vi "AR Example.vi"() -> ()   [LabVIEW 2020]
uses:
  UI_Actor/UI_Actor/ctl_AR_Parameters.ctl
  UI_Actor/UI_Actor/ctl_AR_Mode.ctl
  UIA_ChildTest/UIA_ChildTest/UIA_ChildTest.lvclass
  D:/Projets/STEP AT/UI Actor/UI_Actor/UI_Actor/UI_Actor.lvclass
  UI_Actor/UI_Actor Messages/UI_ShowIn_FreeWindow Msg/UI_ShowIn_FreeWindow Msg.lvclass/UI_ShowIn_FreeWindow Msg.ctl
  UI_Actor/UI_Actor Messages/UI_AutoRefresh Msg/UI_AutoRefresh Msg.lvclass/UI_AutoRefresh Msg.ctl
  support/Actor Framework.lvlibp/Message Enqueuer/Enqueue.vi
  UI_Actor/UI_Actor Messages/UI_ShowIn_FreeWindow Msg/UI_ShowIn_FreeWindow Msg.lvclass
  UI_Actor/UI_Actor Messages/UI_AutoRefresh Msg/UI_AutoRefresh Msg.lvclass
  UI_Actor/UI_Actor/UI_Actor.lvclass
  support/Actor Framework.lvlibp/Stop Msg/Stop Msg.lvclass
  support/Databox.lvlibp
panel:
  in  "Data":dbl[](array[numeric])=[2.0, 2.0, 5.0, 0.0, 0.0, 0.0, 0.0, 3.0, 0.0]
  in  "Parameters":T1={"Write TipStrips with details (T)"=TRUE, "Write Captions with UserLabels (T)"=TRUE, "Mode (ind only)"=enum."Indicators only", "Enable nested stream (T)"=TRUE}
  in  "Units":string[](array[string])=["%", "km", "°C", "-", "", "", " ", "kV", "A"]
  in  "UserLab":string[](array[string])=["coucou 1", "coucou 2", "temp", "c chaud", "", "", " ", "yes!", "Clust num"]
  in  "SysLab":string[](array[string])=["Ctl1", "Ctl2", "indic1", "indic2", "ring", "enum", "slide", "Indic3 in tab ctl", "Clust num"]
  in  "stop":bool
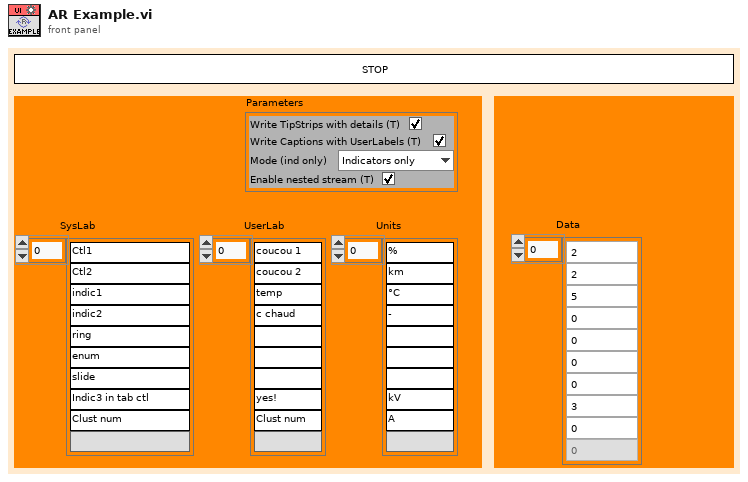
[diagram p1: front panel]
types:
  T1 = typedef "UI_Actor.lvlib/UI_Actor.lvclass/ctl_AR_Parameters.ctl" = cluster{"Write TipStrips with details (T)":bool, "Write Captions with UserLabels (T)":bool, "Mode (ind only)":T2, "Enable nested stream (T)":bool}
  T2 = typedef "UI_Actor.lvlib/UI_Actor.lvclass/ctl_AR_Mode.ctl" = enum16{"Controls only", "Indicators only", "All"}
  T3 = cluster{"Ch.Conf":refnum<class "Config.lvclass">, "Data":refnum<class "Data.lvclass">[]}
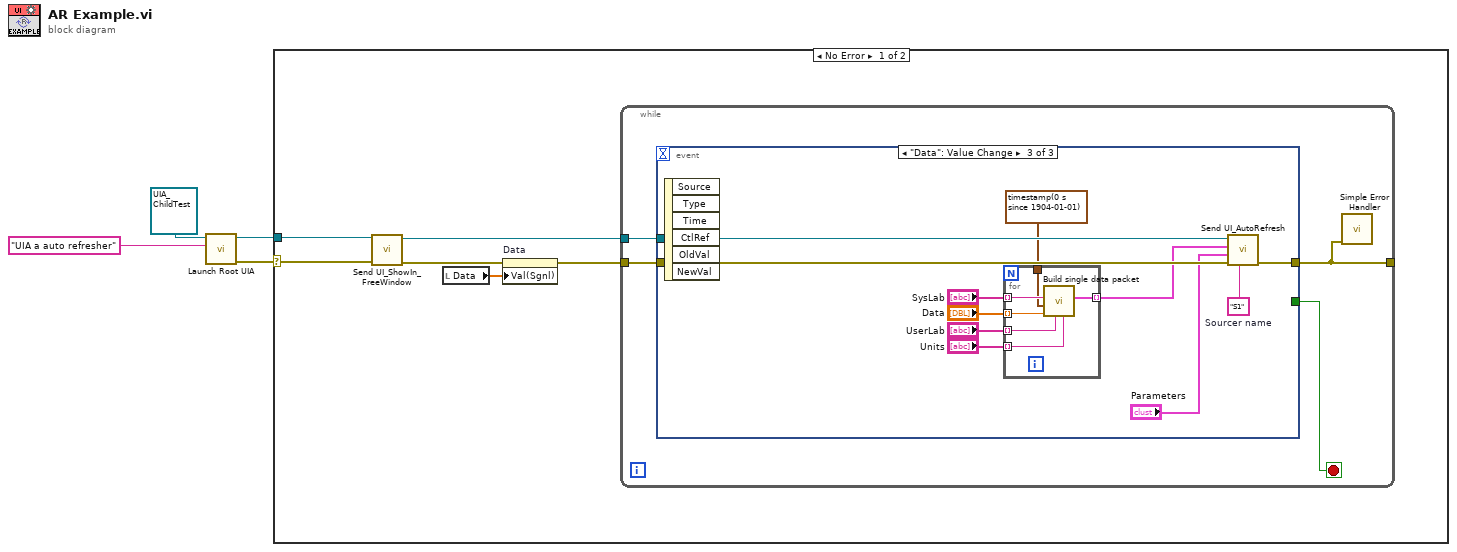
[diagram p0: block diagram]
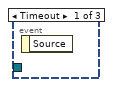
[diagram p2: hidden frame]
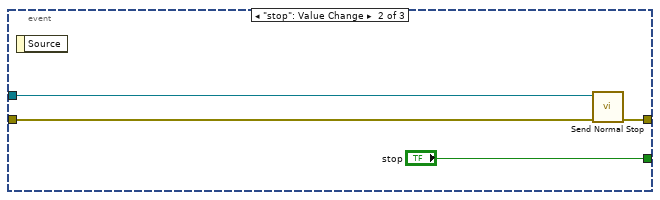
[diagram p3: hidden frame]
diagram:
  n1 = call "Launch Root UIA.vi"("Actor Name"="UIA a auto refresher", "UI_Actor in"=refnum<class "UIA_ChildTest.lvclass"> refnum ("UIA_ChildTest.lvlib:UIA_ChildTest.lvclass")) -> ("error out"=w3:errorcluster, "Actor's Enqueuer"=w4:refnum<class "Message Enqueuer.lvclass">)  [unwired: 8 in]
  n2 = case shown="No Error" w3 {
    selector: w3 -> [w9 _]
    tunnel: w4 -> [w10 _]
    frame No Error {
      n3 = call "Send UI_ShowIn_FreeWindow.vi"("error in (no error)"=w9, "Message Enqueuer"=w10) -> ("error out"=w7:errorcluster, "Message Enqueuer out"=w8:refnum<class "Message Enqueuer.lvclass">)  [unwired: 8 in]
      n4 = local read "Data"() -> (w5:dbl[])
      n5 = property on="Data" class="Arr (strict)"(error in=w7, "Val(Sgnl)"=w5) -> (error out=w6:errorcluster)  [unwired: 1 in, 1 out]
      n6 = while {
        tunnel: w8 -> [w13]
        tunnel: [w11] -> _
        tunnel: w6 -> [w12]
        stop <- w14 stop-if-true
        n7 = event shown="[2] \"Data\": Value Change" {
          selector: _ -> [_ _ _]
          dyn-events: _ -> [_ _ _]
          timeout: _ -> [_ _ _]
          tunnel: [_ "stop" _] -> w14
          tunnel: w13 -> [_ w15 w28]
          tunnel: [_ w16 w27] -> w11
          tunnel: w12 -> [_ w16 w26]
          event Timeout {
            n8 = event-data() -> ()  [unwired: 1 in, 1 out]
          }
          event "stop": Value Change {
            n9 = event-data() -> ()  [unwired: 1 in, 1 out]
            n10 = call "Send Normal Stop.vi"("Message Enqueuer"=w15) -> ()  [unwired: 10 in, 1 out]
          }
          event "Data": Value Change {
            w19 = "S1"  # Sourcer name
            n11 = event-data() -> ()  [unwired: 1 in, 6 out]
            n12 = for {
              tunnel: [w32] -> w24 mode=indexing
              tunnel: "Data" -> [w33] mode=indexing
              tunnel: "SysLab" -> [w34] mode=indexing
              tunnel: "UserLab" -> [w31] mode=indexing
              tunnel: "Units" -> [w30] mode=indexing
              tunnel: timestamp(0 s since 1904-01-01) ("Time (now!)") -> [w29]
              n13 = call "Build single data packet.vi"("Unit"=w30, "User Label"=w31, "Value"=w33, "Time (now!)"=w29, "System Label"=w34) -> ("DataPacket"=w32:T3)  [unwired: 6 in]
            }
            n14 = call "Send UI_AutoRefresh.vi"("Sourcer name"=w19, "error in (no error)"=w26, "Parameters (Tipstrips,Captions,All)"="Parameters", "Data chunk"=w24, "Message Enqueuer"=w28) -> ("error out"=w27:errorcluster)  [unwired: 5 in, 1 out]
          }
        }
        n15 = call <vilib>:"Simple Error Handler.vi"("error in (no error)"=w11) -> ()  [unwired: 4 in, 5 out]
      }
    }
    frame Error {
    }
  }
